vi "INfo_Get.vi"(8 "error in":errorcluster, 10 "select":enum16{"fw", "sn", "pn"}(ring)) -> (0 "error out":errorcluster, 2 "data out":u8[](array[numeric]), 3 "return":i32)   [LabVIEW 2016]
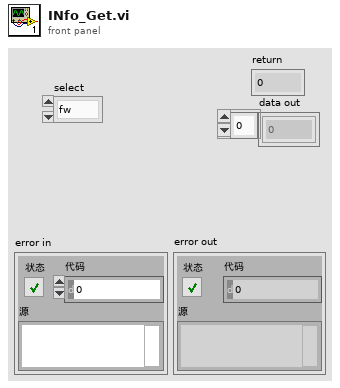
[diagram p1: front panel]
types:
  T1 = cluster{"byCmdType":u8, "bySubCmd":u8, "byPara":u8, "byAddr_h":u8, "byAddr_l":u8, "byAddr_ll":u8, "byLen_h":u8, "byLen_l":u8}
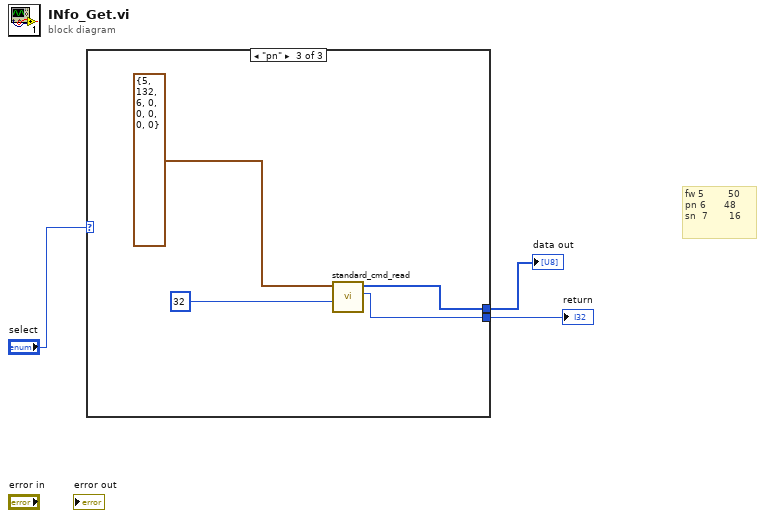
[diagram p0: block diagram]
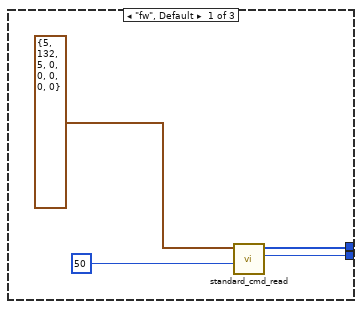
[diagram p2: hidden frame]
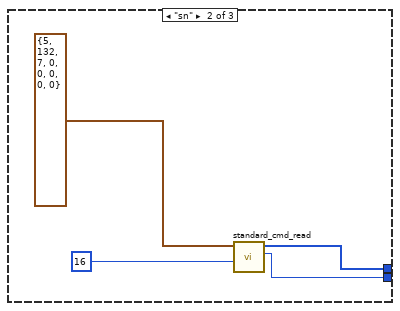
[diagram p3: hidden frame]
diagram:
  # "fw 5        50\npn 6      48\nsn  7       16"
  n1 = case shown="\"pn\"" "select" {
    tunnel: [w5 w9 w13] -> w2
    tunnel: [w4 w8 w12] -> w1
    frame "fw", Default {
      n2 = call "standard_cmd_read.vi"("dwLen"=u32 50, "cmd_std_header_t"=T1 {"byCmdType"=5, "bySubCmd"=132, "byPara"=5, "byAddr_h"=0, "byAddr_l"=0, "byAddr_ll"=0, "byLen_h"=0, "byLen_l"=0}) -> ("return"=w4:i32, "data out"=w5:u8[])  [unwired: 7 in, 1 out]
    }
    frame "sn" {
      n3 = call "standard_cmd_read.vi"("dwLen"=u32 16, "cmd_std_header_t"=T1 {"byCmdType"=5, "bySubCmd"=132, "byPara"=7, "byAddr_h"=0, "byAddr_l"=0, "byAddr_ll"=0, "byLen_h"=0, "byLen_l"=0}) -> ("return"=w8:i32, "data out"=w9:u8[])  [unwired: 7 in, 1 out]
    }
    frame "pn" {
      n4 = call "standard_cmd_read.vi"("dwLen"=u32 32, "cmd_std_header_t"=T1 {"byCmdType"=5, "bySubCmd"=132, "byPara"=6, "byAddr_h"=0, "byAddr_l"=0, "byAddr_ll"=0, "byLen_h"=0, "byLen_l"=0}) -> ("return"=w12:i32, "data out"=w13:u8[])  [unwired: 7 in, 1 out]
    }
  }
  "data out" <- w2
  "return" <- w1
